vi "svc_Check for Equality.vi"(9 "desired precision":dbl=6.0, 10 "n2":dbl format="%0.17f", 11 "n1":dbl format="%0.17f") -> (1 "measured precision":i32, 3 "equal?":bool)   [LabVIEW 2017]
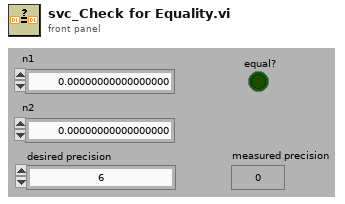
[diagram p1: front panel]
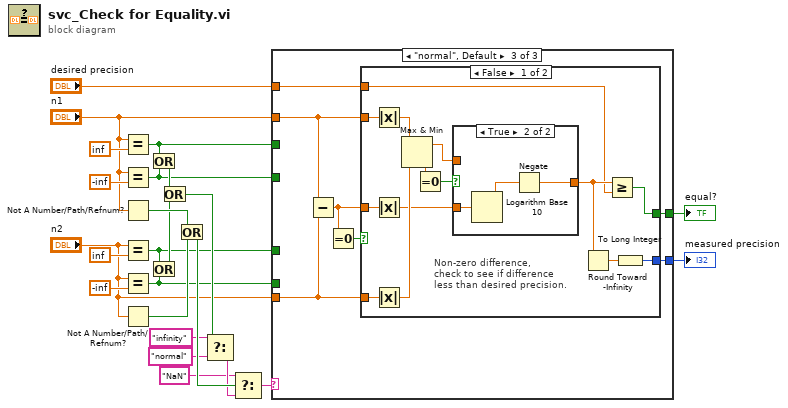
[diagram p0: block diagram]
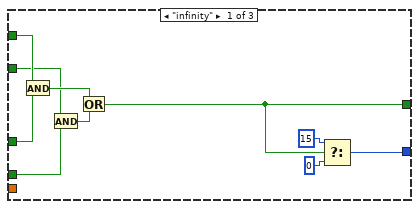
[diagram p2: hidden frame]
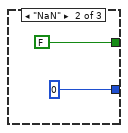
[diagram p3: hidden frame]
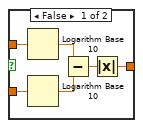
[diagram p4: hidden frame]
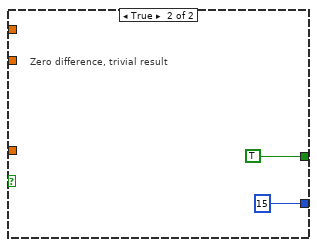
[diagram p5: hidden frame]
diagram:
  n1 = Equal?(x="n1", y=inf ("Positive Infinity")) -> (x = y?=w8:bool)
  n2 = Equal?(x="n1", y=-inf ("Negative Infinity")) -> (x = y?=w9:bool)
  n3 = Not A Number/Path/Refnum?(number/path/refnum="n1") -> (NaN/Path/Refnum?=w20:bool)
  n4 = Equal?(x="n2", y=inf ("Positive Infinity")) -> (x = y?=w7:bool)
  n5 = Equal?(x="n2", y=-inf ("Negative Infinity")) -> (x = y?=w6:bool)
  n6 = Not A Number/Path/Refnum?(number/path/refnum="n2") -> (NaN/Path/Refnum?=w19:bool)
  n7 = Or(x=w8, y=w9) -> (x .or. y?=w18:bool)
  n8 = Or(x=w7, y=w6) -> (x .or. y?=w17:bool)
  n9 = Or(x=w18, y=w17) -> (x .or. y?=w16:bool)
  n10 = Or(x=w20, y=w19) -> (x .or. y?=w15:bool)
  n11 = Select(t="infinity", s=w16, f="normal") -> (s? t:f=w14:string)
  n12 = Select(t="NaN", s=w15, f=w14) -> (s? t:f=w10:string)
  n13 = case shown="\"normal\", Default" w10 {
    tunnel: [w27 FALSE w39] -> w4
    tunnel: [w28 0 w38] -> w3
    tunnel: w9 -> [w29 _ _]
    tunnel: w8 -> [w34 _ _]
    tunnel: w7 -> [w33 _ _]
    tunnel: w6 -> [w30 _ _]
    tunnel: "n1" -> [_ _ w41]
    tunnel: "n2" -> [_ _ w40]
    tunnel: "desired precision" -> [_ _ w37]
    frame "infinity" {
      n14 = And(x=w34, y=w33) -> (x .and. y?=w32:bool)
      n15 = And(x=w29, y=w30) -> (x .and. y?=w31:bool)
      n16 = Or(x=w32, y=w31) -> (x .or. y?=w27:bool)
      n17 = Select(t=15, s=w27, f=0) -> (s? t:f=w28:i32)
    }
    frame "NaN" {
    }
    frame "normal", Default {
      n18 = Subtract(x=w41, y=w40) -> (x-y=w42:dbl)
      n19 = Equal To 0?(x=w42) -> (x = 0?=w43:bool)
      n20 = case shown="False" w43 {
        tunnel: w42 -> [w57 _]
        tunnel: w41 -> [w52 _]
        tunnel: w40 -> [w51 _]
        tunnel: [w54 TRUE] -> w39
        tunnel: [w53 15] -> w38
        tunnel: w37 -> [w44 _]
        frame False {
          # "Non-zero difference,\ncheck to see if difference\nless than desired precision."
          n21 = Absolute Value(x=w52) -> (abs(x)=w50:dbl)
          n22 = Absolute Value(x=w57) -> (abs(x)=w47:dbl)
          n23 = Absolute Value(x=w51) -> (abs(x)=w49:dbl)
          n24 = Max & Min(x=w50, y=w49) -> (max(x,y)=w45:dbl, min(x,y)=w46:dbl)
          n25 = Equal To 0?(x=w46) -> (x = 0?=w48:bool)
          n26 = case shown="True" w48 {
            tunnel: [w58 w64] -> w55
            tunnel: w45 -> [w60 _]
            tunnel: w47 -> [w59 w66]
            frame False {
              n27 = Logarithm Base 10(1:w60) -> (0:w63:dbl)
              n28 = Logarithm Base 10(1:w59) -> (0:w62:dbl)
              n29 = Subtract(x=w63, y=w62) -> (x-y=w61:dbl)
              n30 = Absolute Value(x=w61) -> (abs(x)=w58:dbl)
            }
            frame True {
              n31 = Logarithm Base 10(1:w66) -> (0:w65:dbl)
              n32 = Negate(x=w65) -> (-x=w64:dbl)
            }
          }
          n33 = Round Toward -Infinity ("Round To -Infinity")(1:w55) -> (0:w56:dbl)
          n34 = Greater Or Equal?(x=w55, y=w44) -> (x >= y?=w54:bool)
          n35 = To Long Integer(number=w56) -> (32bit integer=w53:i32)
        }
        frame True {
          # "Zero difference, trivial result"
        }
      }
    }
  }
  "measured precision" <- w3
  "equal?" <- w4
